vi "V2um.vi"(1 "Numeric":dbl, 2 "V2um":dbl=10.0) -> (0 "x*y":dbl)   [LabVIEW 2019]
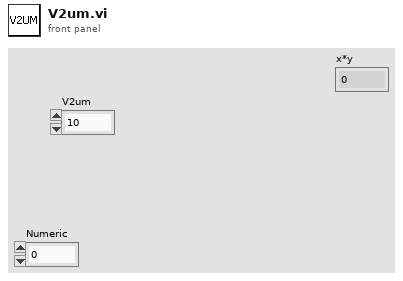
[diagram p1: front panel]
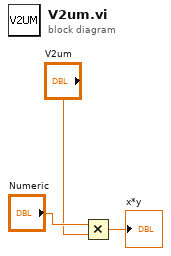
[diagram p0: block diagram]
diagram:
  n1 = Multiply(x="Numeric", y="V2um") -> (x*y=→"x*y":dbl)
